vi "Configure Marker State.vi"(7 "Marker On":bool, 8 "error in (no error)":errorcluster, 10 "Marker Number":u8=1, 11 "VNA-Keysight PNA in":refnum<class "VNA-Keysight PNA.lvclass">) -> (0 "error out":errorcluster, 3 "VNA-Keysight PNA out":refnum<class "VNA-Keysight PNA.lvclass">)   [LabVIEW 2020, in "VNA-Keysight PNA.lvclass"]
doc: "Configure the marker state.\nThe marker is on the active trace."
uses:
  VNA-Keysight PNA.lvclass
  C:/Sandbox/RF Bench/Source Code/WiSpry Test Framework/Instruments/Instrument.lvclass
  Instrument.lvclass/Instrument.ctl
  Instrument.lvclass
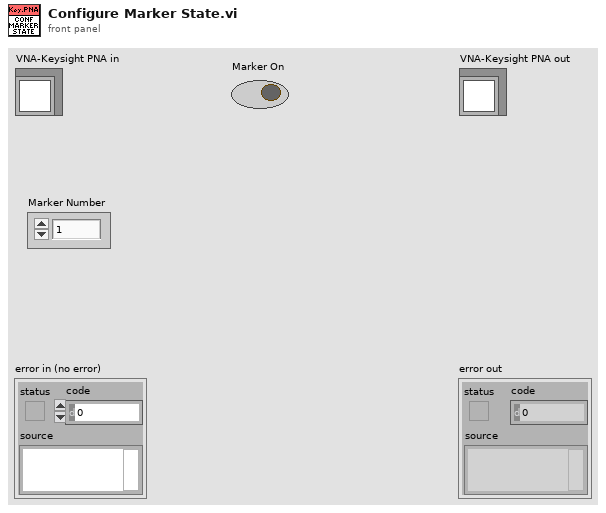
[diagram p1: front panel]
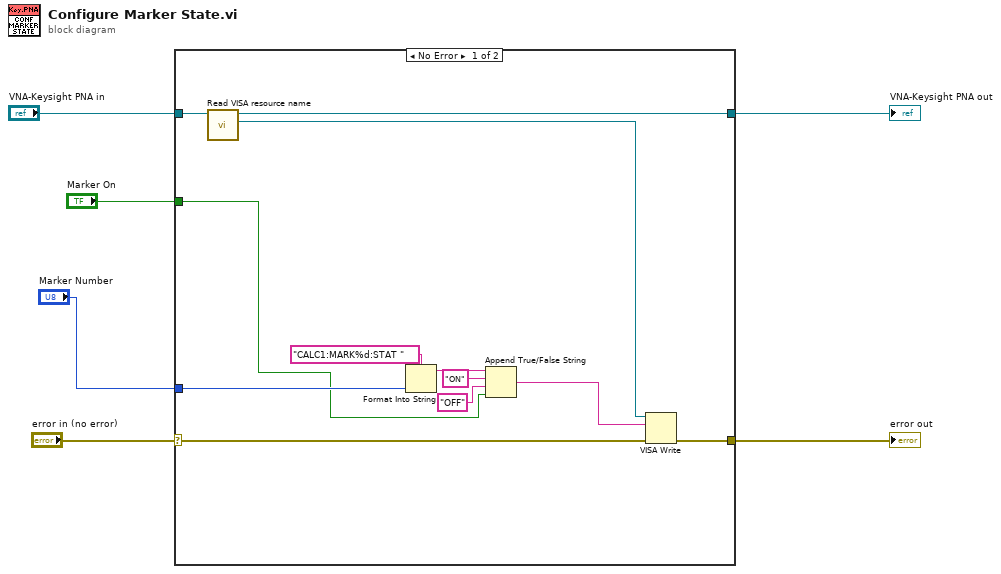
[diagram p0: block diagram]
diagram:
  n1 = case shown="No Error" "error in (no error)" {
    selector: "error in (no error)" -> [w11 w19]
    tunnel: [w17 w20] -> w5
    tunnel: "VNA-Keysight PNA in" -> [w18 w20]
    tunnel: [w10 w19] -> w6
    tunnel: "Marker Number" -> [w8 _]
    tunnel: "Marker On" -> [w7 _]
    frame No Error {
      n2 = call "Read VISA resource name.vi"("Instrument in"=w18) -> ("VISA resource name"=w9:refnum<visa-resource-name>, "Instrument out"=w17:refnum<class "VNA-Keysight PNA.lvclass">)  [unwired: 9 in]
      n3 = Format Into String(format string="CALC1:MARK%d:STAT ", w8) -> (resulting string=w15:string)  [unwired: 2 in, 1 out]
      n4 = Append True/False String(1:w7, 2:"OFF" ("false string"), 3:"ON" ("true string"), 4:w15) -> (0:w12:string)
      n5 = VISA Write(VISA resource name=w9, write buffer=w12, error in (no error)=w11) -> (error out=w10:errorcluster)  [unwired: 2 out]
    }
    frame Error {
    }
  }
  "error out" <- w6
  "VNA-Keysight PNA out" <- w5
